vi "Test Serial 1.vi"() -> ()   [LabVIEW 2014]
uses:
  <vilib>/LabVIEW Universal Transcriptor/LabVIEW to Arduino Transcriptor/Transcriptors/System API/System Serial Library Variables/System Serial Library Variables.lvlib
panel:
  out "data":i32
  out "String Buffer":string
  out "Error Out":errorcluster
  in  "Error In":errorcluster
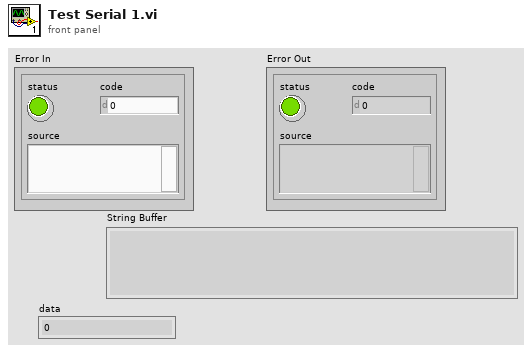
[diagram p1: front panel]
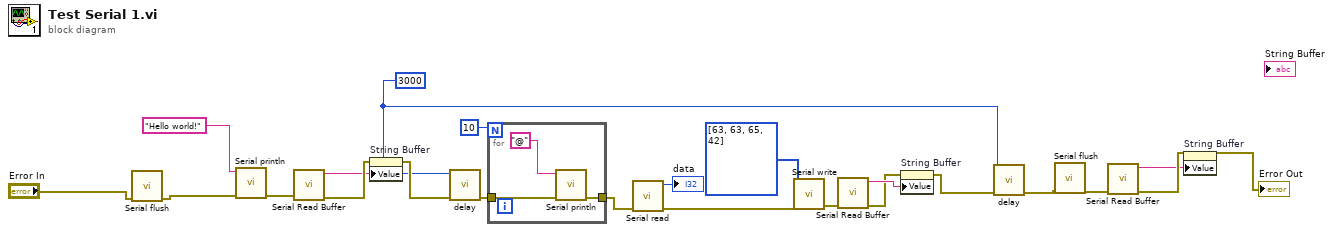
[diagram p0: block diagram]
diagram:
  w16 = 3000 ("time (ms)")
  n1 = call "Serial flush.vi"("Error In"="Error In") -> ("Error Out"=w14:errorcluster)  [unwired: 10 in]
  n2 = call <vilib>:"Serial println.vi"("Error In"=w14, "string in"="Hello world!") -> ("Error Out"=w22:errorcluster)  [unwired: 9 in]
  n3 = call <vilib>:"Serial Read Buffer.vi"("Error In"=w22) -> ("Error Out"=w21:errorcluster, "String Buffer"=w19:string)  [unwired: 9 in]
  n4 = property on="String Buffer" class="Str"(error in=w21, "Value"=w19) -> (error out=w20:errorcluster)  [unwired: 1 in, 1 out]
  n5 = call <vilib>:"delay.vi"("Error In"=w20, "time (ms)"=w16) -> ("Error Out"=w18:errorcluster)  [unwired: 9 in]
  n6 = for {
    N: 10 -> [_]
    tunnel: w18 -> [w26]
    tunnel: [w24] -> w17
    n7 = call <vilib>:"Serial println.vi"("Error In"=w26, "string in"="@") -> ("Error Out"=w24:errorcluster)  [unwired: 9 in]
  }
  n8 = call "Serial read.vi"("Error In"=w17) -> ("Error Out"=w6:errorcluster, "data"=→"data":i32)  [unwired: 9 in]
  n9 = call "Serial write.vi"("Error In"=w6, "bytes[]"=i8[] [63, 63, 65, 42]) -> ("Error Out"=w4:errorcluster)  [unwired: 9 in]
  n10 = call <vilib>:"Serial Read Buffer.vi"("Error In"=w4) -> ("Error Out"=w2:errorcluster, "String Buffer"=w3:string)  [unwired: 9 in]
  n11 = property on="String Buffer" class="Str"(error in=w2, "Value"=w3) -> (error out=w1:errorcluster)  [unwired: 1 in, 1 out]
  n12 = call <vilib>:"delay.vi"("Error In"=w1, "time (ms)"=w16) -> ("Error Out"=w15:errorcluster)  [unwired: 9 in]
  n13 = call "Serial flush.vi"("Error In"=w15) -> ("Error Out"=w9:errorcluster)  [unwired: 10 in]
  n14 = call <vilib>:"Serial Read Buffer.vi"("Error In"=w9) -> ("Error Out"=w12:errorcluster, "String Buffer"=w11:string)  [unwired: 9 in]
  n15 = property on="String Buffer" class="Str"(error in=w12, "Value"=w11) -> (error out=→"Error Out":errorcluster)  [unwired: 1 in, 1 out]
